vi "bindata_descr to JSON.vi"(8 "error in (no error)":errorcluster, 11 "bindata_descriptions":T1[](array[typedef])) -> (0 "error out":errorcluster, 3 "JSON string out":string)   [LabVIEW 2018, in "LV-Julia_ZMQ-Roundtrip_lib.lvlib"]
uses:
  LV-Julia_ZMQ-Roundtrip_lib.lvlib
  Bindata description.ctl
  bindata-only cluster.ctl
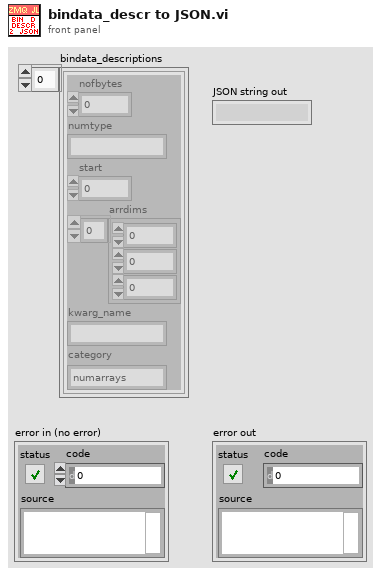
[diagram p1: front panel]
types:
  T1 = typedef "LV-Julia_ZMQ-Roundtrip_lib.lvlib/Bindata description.ctl" = cluster{"nofbytes":i32, "numtype":string, "start":i32, "arrdims":i32[], "kwarg_name":string, "category":string}
  T2 = typedef "LV-Julia_ZMQ-Roundtrip_lib.lvlib/bindata-only cluster.ctl" = cluster{"bindata_descr":T1[]}
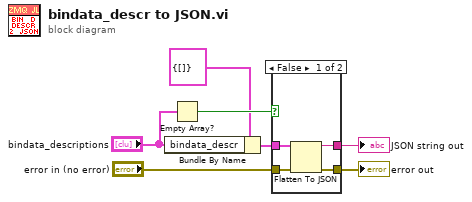
[diagram p0: block diagram]
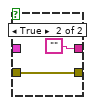
[diagram p2: hidden frame]
diagram:
  n1 = Bundle By Name(cluster=T2 {"bindata_descr"=[]} ("bindata description"), "bindata_descr"="bindata_descriptions") -> (w2:T2)
  n2 = Empty Array?(array="bindata_descriptions") -> (empty?=w4:bool)
  n3 = case shown="False" w4 {
    tunnel: [w9 ""] -> w6
    tunnel: w2 -> [w11 _]
    tunnel: "error in (no error)" -> [w10 w12]
    tunnel: [w8 w12] -> w7
    frame False {
      n4 = Flatten To JSON(anything=w11, error in (no error)=w10) -> (JSON string=w9:string, 11:w8:errorcluster)  [unwired: 1 in]
    }
    frame True {
    }
  }
  "error out" <- w7
  "JSON string out" <- w6
